vi "Update When Mouse Move.vi"(8 "error in (no error)":errorcluster, 10 "Graphic":refnum<class "Graphic.lvclass">, 11 "Canvas in":refnum<class "Canvas.lvclass">) -> (0 "error out":errorcluster, 3 "Canvas out":refnum<class "Canvas.lvclass">)   [LabVIEW 2015, in "Canvas.lvclass"]
uses:
  Canvas.lvclass
  Graphic/Graphic.lvclass
  Canvas.lvclass/Canvas.ctl
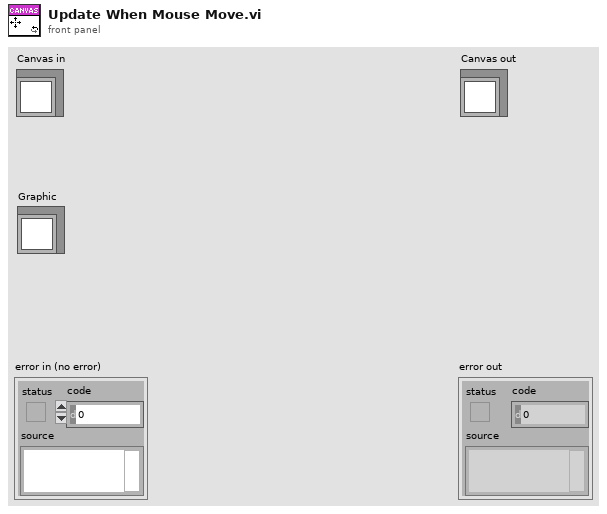
[diagram p1: front panel]
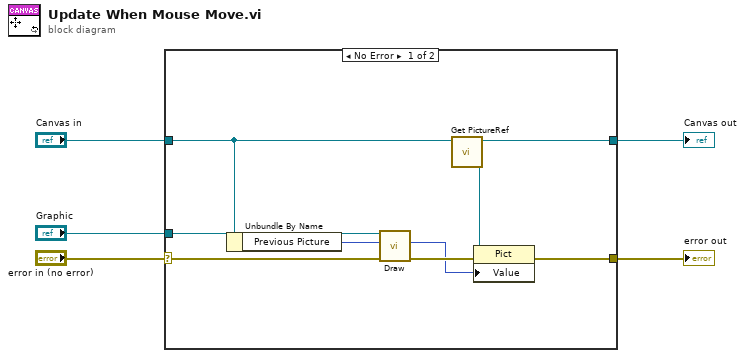
[diagram p0: block diagram]
diagram:
  n1 = case shown="No Error" "error in (no error)" {
    selector: "error in (no error)" -> [w11 w16]
    tunnel: [w10 w16] -> w4
    tunnel: [w13 w15] -> w2
    tunnel: "Canvas in" -> [w14 w15]
    tunnel: "Graphic" -> [w12 _]
    frame No Error {
      n2 = Unbundle By Name(w14) -> ("Previous Picture"=w9:picture)
      n3 = call-dynamic "Draw.vi"("error in (no error)"=w11, "Picture in"=w9, "Graphic in"=w12) -> ("error out"=w8:errorcluster, "Picture out"=w6:picture)  [unwired: 6 in, 1 out]
      n4 = call "Get PictureRef.vi"("Canvas in"=w14) -> ("PictureRef"=w7:refnum<vi>, "Canvas out"=w13:refnum<class "Canvas.lvclass">)  [unwired: 8 in, 1 out]
      n5 = property class="Pict"(reference=w7, error in=w8, "Value"=w6) -> (error out=w10:errorcluster)  [unwired: 1 out]
    }
    frame Error {
    }
  }
  "error out" <- w4
  "Canvas out" <- w2
